vi "Practica9_LedRGB.vi"() -> ()   [LabVIEW 2015]
uses:
  <vilib>/LabVIEW Interface for Arduino/LabVIEW Interface for Arduino.lvlib
panel:
  in  "stop":bool
  in  "Azul":dbl(slide) scale=0.0..255.0
  in  "Verde":dbl(slide) scale=0.0..255.0
  in  "Rojo":dbl(slide) scale=0.0..255.0
  # "LED RGB"
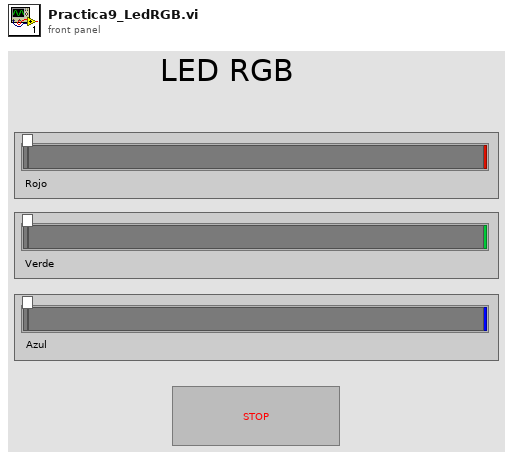
[diagram p1: front panel]
types:
  T1 = typedef "LabVIEW Interface for Arduino.lvlib/Arduino Resource.ctl" = cluster{"VISA resource":refnum<visa-resource-name>, "Board Type":T2, "Connection Type":enum8{"USB / Serial"}, "Bytes Per Packet (15)":u8}
  T2 = typedef "LabVIEW Interface for Arduino.lvlib/Board Type.ctl" = enum16{"Uno", "Dimuelanove w/Atmega 328", "Mega 2560"}
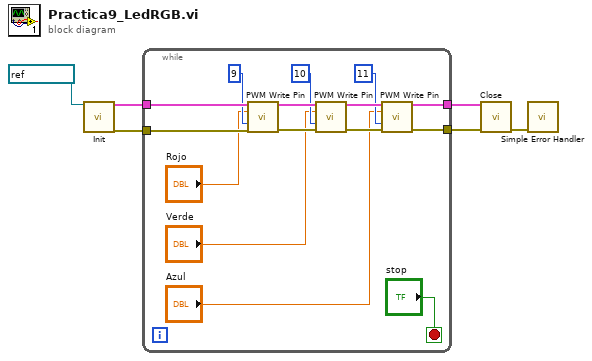
[diagram p0: block diagram]
diagram:
  n1 = call <vilib>:"Init.vi"("VISA resource"=refnum<visa-resource-name> "COM6") -> ("Arduino Resource"=w4:T1, "error out"=w5:errorcluster)  [unwired: 17 in]
  n2 = while {
    tunnel: w5 -> [w21]
    tunnel: w4 -> [w20]
    tunnel: [w15] -> w3
    tunnel: [w14] -> w2
    stop <- "stop" stop-if-true
    n3 = call <vilib>:"PWM Write Pin.vi"("Arduino Resource"=w20, "Duty Cycle (0 - 255)"="Rojo", "PWM Pin (3)"=u8 9, "error in"=w21) -> ("Arduino Resource"=w19:T1, "error out"=w17:errorcluster)  [unwired: 10 in]
    n4 = call <vilib>:"PWM Write Pin.vi"("Arduino Resource"=w19, "Duty Cycle (0 - 255)"="Verde", "PWM Pin (3)"=u8 10, "error in"=w17) -> ("Arduino Resource"=w18:T1, "error out"=w16:errorcluster)  [unwired: 10 in]
    n5 = call <vilib>:"PWM Write Pin.vi"("Arduino Resource"=w18, "Duty Cycle (0 - 255)"="Azul", "PWM Pin (3)"=u8 11, "error in"=w16) -> ("Arduino Resource"=w14:T1, "error out"=w15:errorcluster)  [unwired: 10 in]
  }
  n6 = call <vilib>:"Close.vi"("Arduino Resource"=w2, "error in"=w3) -> ("error out"=w1:errorcluster)  [unwired: 13 in]
  n7 = call <vilib>:"Simple Error Handler.vi"("error in (no error)"=w1) -> ()  [unwired: 4 in, 5 out]
